vi "Modbus Slave.vi"(0 "Modbus Status Interface Data":T2 {"GenEast"."DefLevel" format="%04x"; "GenEast"."BatteryVoltage" format="%04x"; "GenEast"."Frequency" format="%04x"; "GenEast"."PowerFactor" format="%04x"; "GenEast"."ControllerMode" format="%04x"; "GenEast"."TotalFuel" format="%04x"; "GenEast"."FuelRate" format="%04x"; "GenEast"."ApparentPower" format="%04x"; "GenEast"."RunHours" format="%04x"; "GenEast"."ReactivePower" format="%04x"; "GenEast"."ActivePower" format="%04x"; "GenEast"."Alarms" format="%04x"; "GenWest"."DefLevel" format="%04x"; "GenWest"."BatteryVoltage" format="%04x"; "GenWest"."Frequency" format="%04x"; "GenWest"."PowerFactor" format="%04x"; "GenWest"."ControllerMode" format="%04x"; "GenWest"."TotalFuel" format="%04x"; "GenWest"."FuelRate" format="%04x"; "GenWest"."ApparentPower" format="%04x"; "GenWest"."RunHours" format="%04x"; "GenWest"."ReactivePower" format="%04x"; "GenWest"."ActivePower" format="%04x"; "GenWest"."Alarms" format="%04x"; "Converter Alarms 2" format="%016b"; "Converter Faults 2" format="%016b"; "Controller Faults" format="%016b"; "System Status" format="%016b"; "Converter Alarms 1" format="%016b"; "Converter Faults 1" format="%016b"; "Solar Faults" format="%016b"; "ES Rack 10 Alarms" format="%016b"; "ES Rack 9 Alarms" format="%016b"; "ES Rack 8 Alarms" format="%016b"; "ES Rack 7 Alarms" format="%016b"; "ES Rack 6 Alarms" format="%016b"; "ES Rack 5 Alarms" format="%016b"; "ES Rack 4 Alarms" format="%016b"; "ES Rack 3 Alarms" format="%016b"; "ES Rack 2 Alarms" format="%016b"; "ES Rack 1 Alarms" format="%016b"; "ES System Alarms" format="%016b"; "System Faults" format="%016b"; "ES Rack 10 Faults" format="%016b"; "ES Rack 9 Faults" format="%016b"; "ES Rack 8 Faults" format="%016b"; "ES Rack 7  Faults" format="%016b"; "ES Rack 6 Faults" format="%016b"; "ES Rack 5 Faults" format="%016b"; "ES Rack 4 Faults" format="%016b"; "ES Rack 3 Faults" format="%016b"; "ES Rack 2 Faults" format="%016b"; "ES Rack 1 Faults" format="%016b"; "ES System Faults" format="%016b"}, 11 "Error In":errorcluster) -> (4 "TCP Connection Count":u32, 6 "TCP Connection List":T1(array[cluster]), 15 "Error Out":errorcluster)   [LabVIEW 2014]
uses:
  Controls/ModbusState.ctl
  <vilib>/Modbus/slave/Modbus Slave.lvclass
  <vilib>/Modbus/slave/Create Slave Instance (TCP).vi
  Controls/Interface Data.ctl
  Controls/Gen Data.ctl
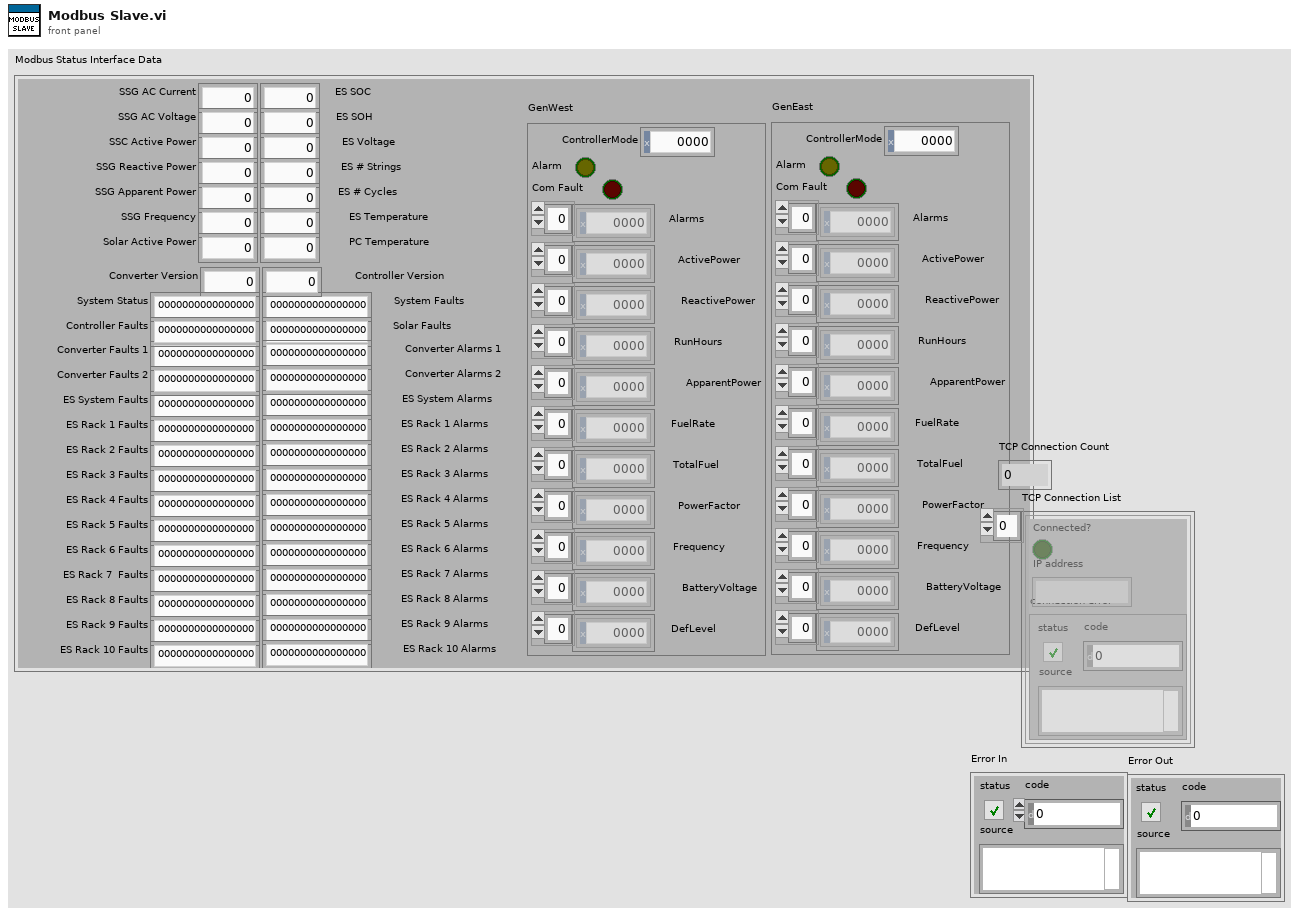
[diagram p1: front panel]
types:
  T1 = cluster{"Connected?":bool, "IP address":string, "connection error":errorcluster}[]
  T2 = typedef "Interface Data.ctl" = cluster{"SSG AC Current":i16, "SSG AC Voltage":i16, "SSC Active Power":i16, "SSG Reactive Power":i16, "SSG Apparent Power":i16, "SSG Frequency":i16, "ES SOC":i16, "ES SOH":i16, "ES Voltage":i16, "ES # Strings":i16, "ES # Cycles":i16, "ES Temperature":i16, "PC Temperature":i16, "Solar Active Power":i16, "Converter Version":i16, "Controller Version":i16, "System Status":i16, "System Faults":i16, "Controller Faults":i16, "ES System Faults":i16, "ES System Alarms":i16, "Converter Faults 1":i16, "Converter Faults 2":i16, "Converter Alarms 1":i16, "Converter Alarms 2":i16, "Solar Faults":i16, "ES Rack 1 Faults":i16, "ES Rack 2 Faults":i16, "ES Rack 3 Faults":i16, "ES Rack 4 Faults":i16, "ES Rack 5 Faults":i16, "ES Rack 6 Faults":i16, "ES Rack 7  Faults":i16, "ES Rack 8 Faults":i16, "ES Rack 9 Faults":i16, "ES Rack 10 Faults":i16, "ES Rack 1 Alarms":i16, "ES Rack 2 Alarms":i16, "ES Rack 3 Alarms":i16, "ES Rack 4 Alarms":i16, "ES Rack 5 Alarms":i16, "ES Rack 6 Alarms":i16, "ES Rack 7 Alarms":i16, "ES Rack 8 Alarms":i16, "ES Rack 9 Alarms":i16, "ES Rack 10 Alarms":i16, "GenWest":T3, "GenEast":T3}
  T3 = typedef "Gen Data.ctl" = cluster{"ControllerMode":u16, "Alarm":bool, "Com Fault":bool, "Alarms":u16[], "ActivePower":u16[], "ReactivePower":u16[], "RunHours":u16[], "ApparentPower":u16[], "FuelRate":u16[], "TotalFuel":u16[], "PowerFactor":u16[], "Frequency":u16[], "BatteryVoltage":u16[], "DefLevel":u16[]}
  T4 = typedef "ModbusState.ctl" = enum16{"Connect", "Disconnect", "Set Basic Objects", "Get Basic Objects", "Read", "Write", "Read/Write"}
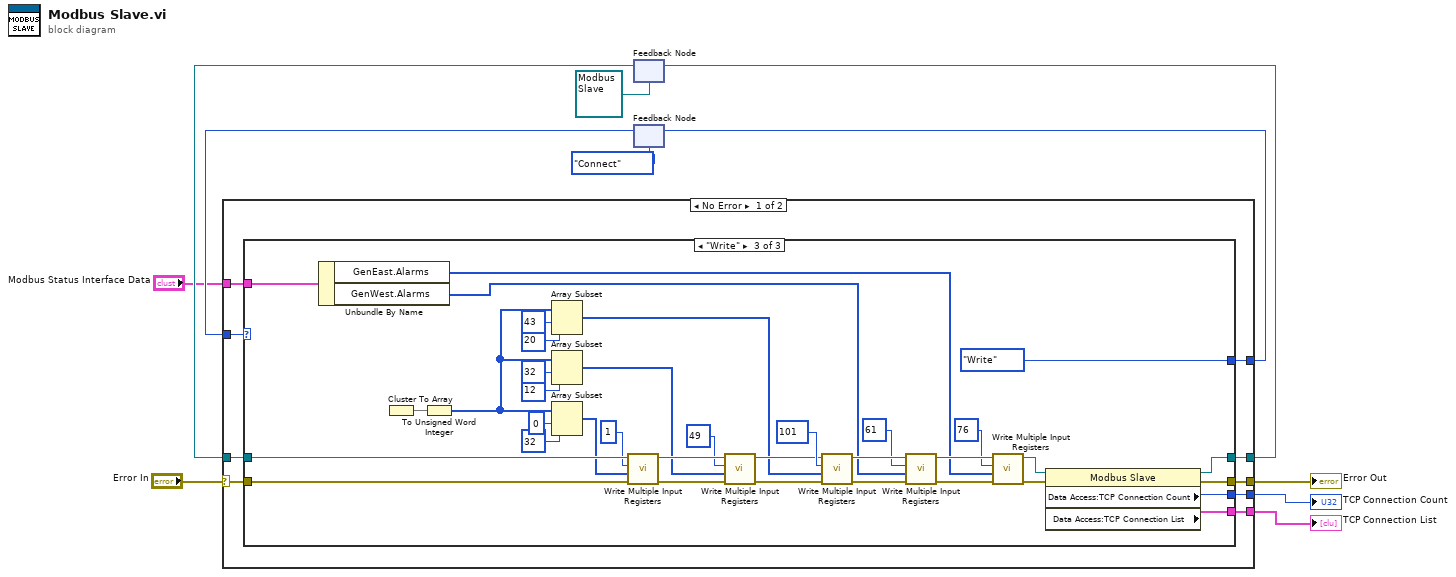
[diagram p0: block diagram]
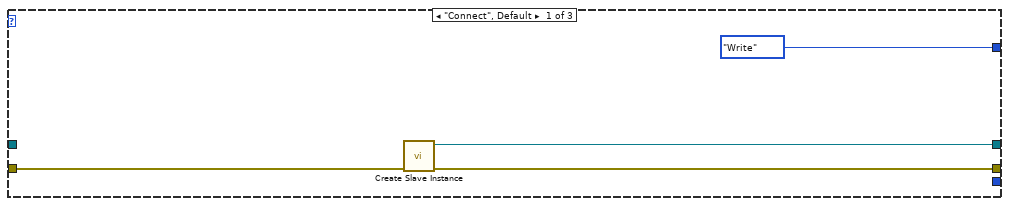
[diagram p2: hidden frame]
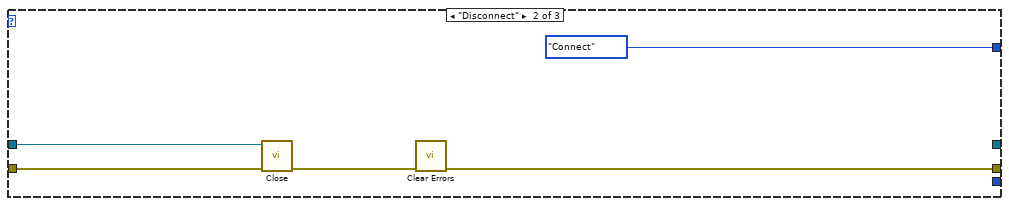
[diagram p3: hidden frame]
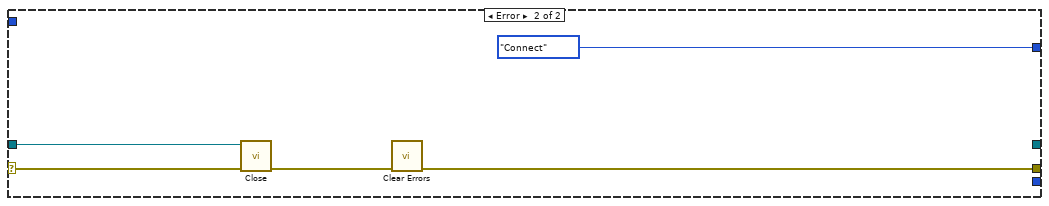
[diagram p4: hidden frame]
diagram:
  n1 = feedback #1(refnum<class "Modbus Slave.lvclass"> refnum ("Modbus slave out")) -> (w6:refnum<class "Modbus Slave.lvclass">)
  n2 = feedback #2(ModbusState."Connect" ("Modbus State")) -> (w7:T4)
  n3 = case shown="No Error" "Error In" {
    selector: "Error In" -> [w19 w69]
    tunnel: w7 -> [w20 _]
    tunnel: [w16 w68] -> w10
    tunnel: [w18 _] -> w5
    tunnel: [w17 ModbusState."Connect" ("Modbus State")] -> w9
    tunnel: w6 -> [w15 w67]
    tunnel: "Modbus Status Interface Data" -> [w14 _]
    tunnel: [w13 _] -> w2
    tunnel: [w12 _] -> w1
    frame No Error {
      n4 = case shown="\"Write\"" w20 {
        tunnel: w19 -> [w21 w29 w59]
        tunnel: [w23 _ w35] -> w18
        tunnel: [ModbusState."Write" ("Modbus State") ModbusState."Connect" ("Modbus State") ModbusState."Write" ("Modbus State")] -> w17
        tunnel: [w24 w28 w36] -> w16
        tunnel: w15 -> [_ w26 w64]
        tunnel: w14 -> [_ _ w32]
        tunnel: [_ _ w34] -> w13
        tunnel: [_ _ w33] -> w12
        frame "Connect", Default {
          n5 = call-poly <vilib>:"Create Slave Instance.vi"("error in (no error)"=w21) -> ("error out"=w24:errorcluster, "TCP slave instance"=w23:refnum<class "Modbus Slave.lvclass">)  [unwired: 9 in]
        }
        frame "Disconnect" {
          n6 = call-dynamic "Close.vi"("error in (no error)"=w29, "Modbus slave in"=w26) -> ("error out"=w25:errorcluster)  [unwired: 9 in]
          n7 = call <vilib>:"Clear Errors.vi"("error in (no error)"=w25) -> ("error out"=w28:errorcluster)  [unwired: 5 in, 1 out]
        }
        frame "Write" {
          n8 = Unbundle By Name(w32) -> ("GenEast.Alarms"=w31:u16[], "GenWest.Alarms"=w30:u16[])
          n9 = Cluster To Array() -> (array=w55:void[])  [unwired: 1 in]
          n10 = To Unsigned Word Integer(number=w55) -> (unsigned 16bit integer=w49:u16[])
          n11 = Array Subset(array=w49, index=43, length=20) -> (w45:u16[])
          n12 = Array Subset(array=w49, index=32, length=12) -> (w46:u16[])
          n13 = Array Subset(array=w49, index=0, length=32) -> (w52:u16[])
          n14 = call-dynamic "Write Multiple Input Registers.vi"("error in (no error)"=w59, "input register values"=w52, "starting address"=u16 1, "Modbus slave in"=w64) -> ("error out"=w60:errorcluster, "Modbus slave out"=w63:refnum<class "Modbus Slave.lvclass">)  [unwired: 6 in]
          n15 = call-dynamic "Write Multiple Input Registers.vi"("error in (no error)"=w60, "input register values"=w46, "starting address"=u16 49, "Modbus slave in"=w63) -> ("error out"=w61:errorcluster, "Modbus slave out"=w62:refnum<class "Modbus Slave.lvclass">)  [unwired: 6 in]
          n16 = call-dynamic "Write Multiple Input Registers.vi"("error in (no error)"=w61, "input register values"=w45, "starting address"=u16 101, "Modbus slave in"=w62) -> ("error out"=w44:errorcluster, "Modbus slave out"=w41:refnum<class "Modbus Slave.lvclass">)  [unwired: 6 in]
          n17 = call-dynamic "Write Multiple Input Registers.vi"("error in (no error)"=w44, "input register values"=w30, "starting address"=u16 61, "Modbus slave in"=w41) -> ("error out"=w43:errorcluster, "Modbus slave out"=w42:refnum<class "Modbus Slave.lvclass">)  [unwired: 6 in]
          n18 = call-dynamic "Write Multiple Input Registers.vi"("error in (no error)"=w43, "input register values"=w31, "starting address"=u16 76, "Modbus slave in"=w42) -> ("error out"=w37:errorcluster, "Modbus slave out"=w38:refnum<class "Modbus Slave.lvclass">)  [unwired: 6 in]
          n19 = property class="Modbus Slave"(reference=w38, error in=w37) -> (reference out=w35:refnum<class "Modbus Slave.lvclass">, error out=w36:errorcluster, "Data Access:TCP Connection Count"=w33:u32, "Data Access:TCP Connection List"=w34:T1)
        }
      }
    }
    frame Error {
      n20 = call-dynamic "Close.vi"("error in (no error)"=w69, "Modbus slave in"=w67) -> ("error out"=w66:errorcluster)  [unwired: 9 in]
      n21 = call <vilib>:"Clear Errors.vi"("error in (no error)"=w66) -> ("error out"=w68:errorcluster)  [unwired: 5 in, 1 out]
    }
  }
  "Error Out" <- w10
  "TCP Connection List" <- w2
  "TCP Connection Count" <- w1
  n22 = feedback-in #1(w5) -> ()
  n23 = feedback-in #2(w9) -> ()
